vi "ClientSrv Remote File Dialog.vi"(7 "prompt":string, 8 "pattern":string(combo), 11 "start path":path) -> (0 "cancelled":bool, 2 "path":path)   [LabVIEW 2012]
doc: "A file dialog for selecting a file on the remote server. Can be called as a subVI similar to the standard \"File Dialog\" function."
uses:
  served/ClientSrv Server File Manipulation_srv.ctl
  typedefs/t_ClientSrv Remote File Dialog States.ctl
  typedefs/t_ClientSrv Tree Controller Methods.ctl
panel:
  out "file manipulation":T1
  out "file":string
  in  "cancel":bool
  in  "select":bool
  in  "tree":string(tree)
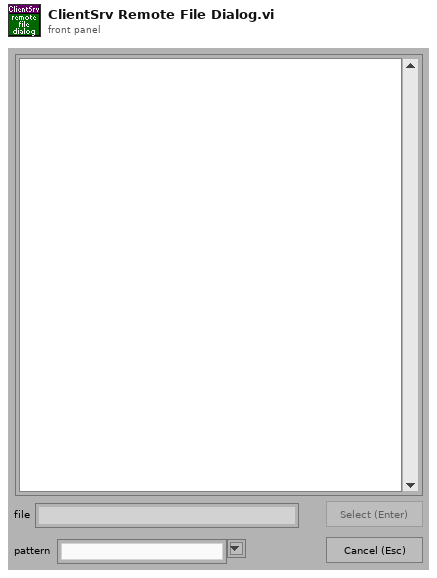
[diagram p1: front panel]
types:
  T1 = typedef "ClientSrv Server File Manipulation_srv.ctl" = refnum<vi>
  T2 = typedef "t_ClientSrv Remote File Dialog States.ctl" = enum16{"empty queue", "initialize", "update tree", "update selected", "persist", "cleanup", "stop"}
  T3 = typedef "t_ClientSrv Tree Controller Methods.ctl" = enum16{"do nothing", "initialize", "open item", "close item", "refresh"}
  T4 = typedef "eventvkey.ctl" = enum16{"ASCII", "Enter", "Return", "Shift", "Ctrl", "Alt", "Cmd", "Opt", "Caps", "NumLock", "Clear", "Break", "Up", "Down", "Left", "Right", "Insert", "Delete", "Home", "End", "PageUp", "PageDown", "Escape", "Help", "Pause", "ScrollLock", "F1", "F2", "F3", "F4", "F5", "F6", "F7", "F8", "F9", "F10", "F11", "F12", "F13", "F14", "F15", "F16", "F17", "F18", "F19", "F20", "F21", "F22", "F23", "F24", "Play", "VolumeUp", "VolumeDown", "Mute", "Two Byte Char"}
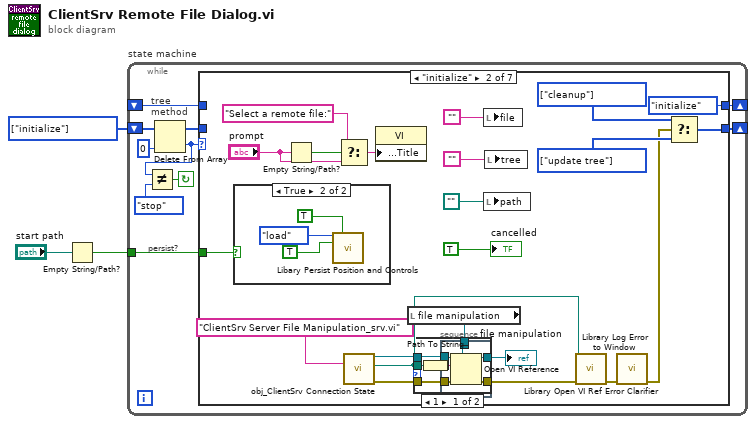
[diagram p0: block diagram]
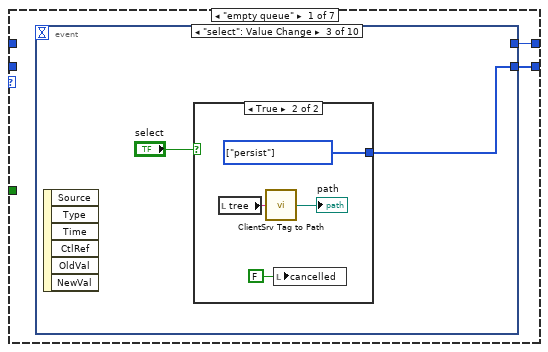
[diagram p2: hidden frame]
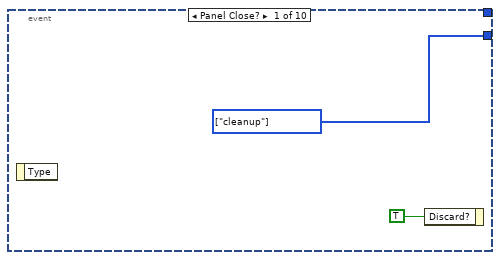
[diagram p3: hidden frame]
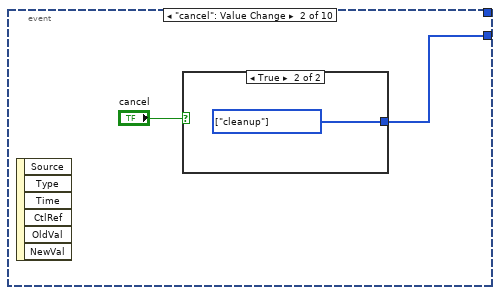
[diagram p4: hidden frame]
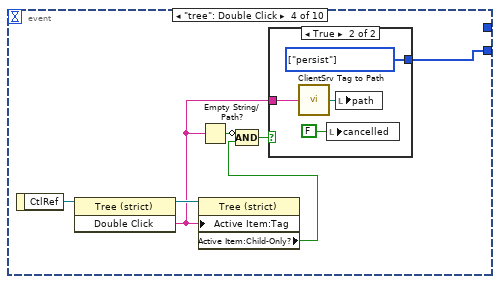
[diagram p7: hidden frame]
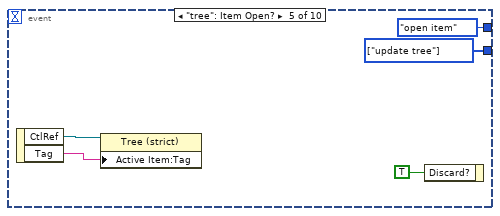
[diagram p9: hidden frame]
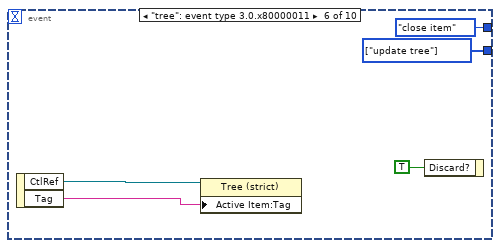
[diagram p10: hidden frame]
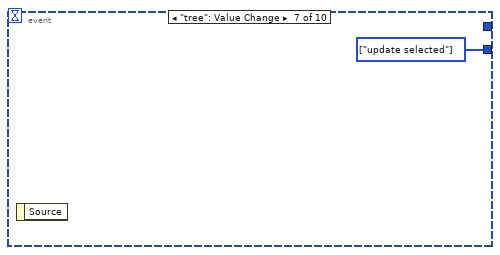
[diagram p11: hidden frame]
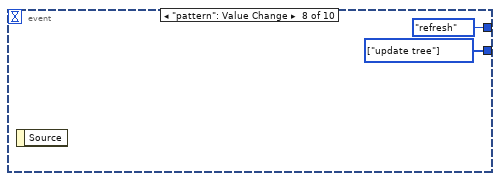
[diagram p12: hidden frame]
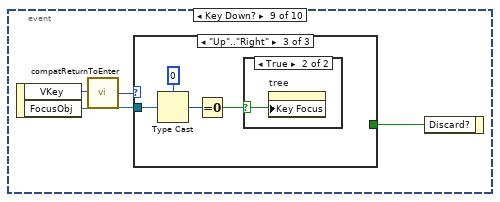
[diagram p13: hidden frame]
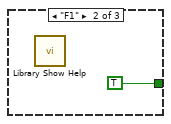
[diagram p15: hidden frame]
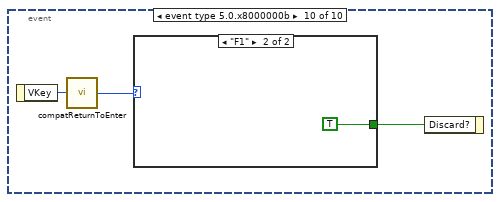
[diagram p17: hidden frame]
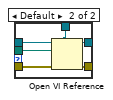
[diagram p19: hidden frame]
diagram:
  w3 = T2[] [enum."initialize"] items=["empty queue", "initialize", "update tree", "update selected", "persist", "cleanup", "stop"] ("Array Constant")
  n1 = Empty String/Path?(string/path="start path") -> (empty?=w1:bool)
  n2 = while "state machine" {
    shift-left: w3 -> [w10]
    shift-right: [w13] -> _
    shift-right: [w5] -> _
    shift-left: _ -> [w6]
    tunnel: w1 -> [w4]
    stop <- w12 continue-if-true
    # "persist?"
    # "tree\nmethod"
    n3 = Delete From Array(array=w10, index=0) -> (deleted portion=w8:T2, array with subset deleted=w9:T2[])  [unwired: 1 in]
    n4 = Not Equal?(x=w8, y=t_ClientSrv_Remote_File_Dialog_States."stop" ("states")) -> (x != y?=w12:bool)
    n5 = case "Case" shown="\"initialize\"" w8 {
      tunnel: [w15 w75 w112 w129 w137 w150 w152] -> w13
      tunnel: w9 -> [_ _ w114 w129 w139 _ w152]
      tunnel: w6 -> [_ _ w113 w128 w138 w149 w151]
      tunnel: [w14 t_ClientSrv_Tree_Controller_Methods."initialize" ("method") w113 w128 w138 w149 w151] -> w5
      tunnel: w4 -> [_ w71 _ _ w135 _ _]
      frame "empty queue" {
        n6 = event shown="[2] \"select\": Value Change" {
          selector: _ -> [_ _ _ _ _ _ _ _ _ _]
          dyn-events: _ -> [_ _ _ _ _ _ _ _ _ _]
          timeout: _ -> [_ _ _ _ _ _ _ _ _ _]
          tunnel: [w17 w19 w22 w29 w42 w45 w48 w49 _ _] -> w15
          tunnel: [_ _ _ _ t_ClientSrv_Tree_Controller_Methods."open item" ("method") t_ClientSrv_Tree_Controller_Methods."close item" ("method") _ t_ClientSrv_Tree_Controller_Methods."refresh" ("method") _ _] -> w14
          event Panel Close? {
            w17 = T2[] [enum."cleanup"] items=["empty queue", "initialize", "update tree", "update selected", "persist", "cleanup", "stop"] ("Array Constant")
            n7 = event-data() -> ()  [unwired: 1 in, 1 out]
            n8 = event-data("Discard?"=TRUE) -> ()  [unwired: 1 in, 1 out]
          }
          event "cancel": Value Change {
            n9 = event-data() -> ()  [unwired: 1 in, 6 out]
            n10 = case shown="True" "cancel" {
              tunnel: [_ w20] -> w19
              frame False {
              }
              frame True {
                w20 = T2[] [enum."cleanup"] items=["empty queue", "initialize", "update tree", "update selected", "persist", "cleanup", "stop"] ("Array Constant")
              }
            }
          }
          event "select": Value Change {
            n11 = event-data() -> ()  [unwired: 1 in, 6 out]
            n12 = case shown="True" "select" {
              tunnel: [_ w26] -> w22
              frame False {
              }
              frame True {
                w26 = T2[] [enum."persist"] items=["empty queue", "initialize", "update tree", "update selected", "persist", "cleanup", "stop"] ("Array Constant")
                n13 = local read "tree"() -> (w25:string)
                n14 = call "ClientSrv Tag to Path.vi"("tree tag"=w25) -> ("path"=→"path":path)
                n15 = local write "cancelled"(FALSE ("cancelled")) -> ()
              }
            }
          }
          event "tree": Double Click {
            n16 = event-data() -> ("CtlRef"=w33:refnum<vi>)  [unwired: 1 in]
            n17 = invoke class="Tree (strict)" method="Double Click"(reference=w33) -> (reference out=w32:refnum<vi>, "Double Click"=w27:string)  [unwired: 2 in, 1 out]
            n18 = property class="Tree (strict)"(reference=w32, "Active Item:Tag"=w27) -> ("Active Item:Child-Only?"=w28:bool)  [unwired: 1 in, 2 out]
            n19 = Empty String/Path?(string/path=w27) -> (empty?=w31:bool)
            n20 = Compound Arithmetic op=AND(invert w31, w28) -> (w30:bool)
            n21 = case shown="True" w30 {
              tunnel: w27 -> [_ w36]
              tunnel: [_ w35] -> w29
              frame False {
              }
              frame True {
                w35 = T2[] [enum."persist"] items=["empty queue", "initialize", "update tree", "update selected", "persist", "cleanup", "stop"] ("Array Constant")
                n22 = call "ClientSrv Tag to Path.vi"("tree tag"=w36) -> ("path"=w37:path)
                n23 = local write "cancelled"(FALSE ("cancelled")) -> ()
                n24 = local write "path"(w37) -> ()
              }
            }
          }
          event "tree": Item Open? {
            w42 = T2[] [enum."update tree"] items=["empty queue", "initialize", "update tree", "update selected", "persist", "cleanup", "stop"] ("Array Constant")
            n25 = event-data() -> ("CtlRef"=w41:refnum<vi>, "Tag"=w40:string)  [unwired: 1 in]
            n26 = property class="Tree (strict)"(reference=w41, "Active Item:Tag"=w40) -> ()  [unwired: 1 in, 2 out]
            n27 = event-data("Discard?"=TRUE) -> ()  [unwired: 1 in, 1 out]
          }
          event "tree": event type 3.0.x80000011 {
            w45 = T2[] [enum."update tree"] items=["empty queue", "initialize", "update tree", "update selected", "persist", "cleanup", "stop"] ("Array Constant")
            n28 = event-data() -> ("CtlRef"=w47:refnum<vi>, "Tag"=w46:string)  [unwired: 1 in]
            n29 = property class="Tree (strict)"(reference=w47, "Active Item:Tag"=w46) -> ()  [unwired: 1 in, 2 out]
            n30 = event-data("Discard?"=TRUE) -> ()  [unwired: 1 in, 1 out]
          }
          event "tree": Value Change {
            w48 = T2[] [enum."update selected"] items=["empty queue", "initialize", "update tree", "update selected", "persist", "cleanup", "stop"] ("Array Constant")
            n31 = event-data() -> ()  [unwired: 1 in, 1 out]
          }
          event "pattern": Value Change {
            w49 = T2[] [enum."update tree"] items=["empty queue", "initialize", "update tree", "update selected", "persist", "cleanup", "stop"] ("Array Constant")
            n32 = event-data() -> ()  [unwired: 1 in, 1 out]
          }
          event Key Down? {
            n33 = event-data() -> ("VKey"=w51:T4, "FocusObj"=w52:refnum<vi>)  [unwired: 1 in]
            n34 = call <vilib>:"compatReturnToEnter.vi"("VKey"=w51) -> ("VKey"=w54:T4)
            n35 = case shown="\"Up\"..\"Right\"" w54 {
              tunnel: [_ TRUE _] -> w53
              tunnel: w52 -> [_ _ w57]
              frame Default {
              }
              frame "F1" {
                n36 = call "Library Show Help.vi"() -> ()  [unwired: 1 in]
              }
              frame "Up".."Right" {
                n37 = Type Cast(type=0, x=w57) -> (*(type *) &x=w59:i32)
                n38 = Equal To 0?(x=w59) -> (x = 0?=w56:bool)
                n39 = case shown="True" w56 {
                  selector: w56 -> [_ w60]
                  frame False {
                  }
                  frame True {
                    n40 = property on="tree" class="Tree (strict)"("Key Focus"=w60) -> ()  [unwired: 2 in, 2 out]
                  }
                }
              }
            }
            n41 = event-data("Discard?"=w53) -> ()  [unwired: 1 in, 1 out]
          }
          event event type 5.0.x8000000b {
            n42 = event-data() -> ("VKey"=w61:T4)  [unwired: 1 in]
            n43 = call <vilib>:"compatReturnToEnter.vi"("VKey"=w61) -> ("VKey"=w63:T4)
            n44 = case shown="\"F1\"" w63 {
              tunnel: [_ TRUE] -> w62
              frame Default {
              }
              frame "F1" {
              }
            }
            n45 = event-data("Discard?"=w62) -> ()  [unwired: 1 in, 1 out]
          }
        }
      }
      frame "initialize" {
        w74 = T2[] [enum."cleanup"] items=["empty queue", "initialize", "update tree", "update selected", "persist", "cleanup", "stop"] ("Array Constant")
        w73 = T2[] [enum."update tree"] items=["empty queue", "initialize", "update tree", "update selected", "persist", "cleanup", "stop"] ("Array Constant")
        n46 = case shown="True" w71 {
          frame False {
          }
          frame True {
            n47 = call "Libary Persist Position and Controls.vi"("action"=enum16{"save", "load"}."load", "do not open (false)"=TRUE, "do not persist bounds (false)"=TRUE) -> ()  [unwired: 11 in, 2 out]
          }
        }
        n48 = Empty String/Path?(string/path="prompt") -> (empty?=w81:bool)
        n49 = Select(t="Select a remote file:", s=w81, f="prompt") -> (s? t:f=w78:string)
        n50 = call "obj_ClientSrv Connection State.vi"("machine{connect}/VI{get state} name (local/no path resolution)"="ClientSrv Server File Manipulation_srv.vi") -> ("server app ref"=w66:refnum<vi>, "resolved server path"=w65:path, "error out"=w70:errorcluster)  [unwired: 7 in, 5 out]
        n51 = property class="VI"("Front Panel Window:Title"=w78) -> ()  [unwired: 2 in, 2 out]
        n52 = local read "file manipulation"() -> (w67:T1)
        n53 = stacked-sequence {
          tunnel: [w92] -> w68
          tunnel: [w91] -> w69
          tunnel: w70 -> [w90]
          tunnel: w66 -> [w89]
          tunnel: w65 -> [w88]
          tunnel: w67 -> [w87]
          frame #0 {
            # "avoid LV8 complaints"
            n54 = Path to Array of Strings(0:w88) -> (2:w93:string[])  [unwired: 1 out]
            n55 = Array Size(array=w93) -> (size(s)=w94:i32)
            n56 = case shown="1" w94 {
              tunnel: w88 -> [w101 w107]
              tunnel: w89 -> [w99 w106]
              tunnel: [w97 w102] -> w92
              tunnel: [w95 w105] -> w91
              tunnel: w87 -> [w96 w104]
              tunnel: w90 -> [w98 w103]
              frame 1 {
                n57 = Path To String(path=w101) -> (string=w100:string)
                n58 = Open VI Reference(type specifier VI Refnum (for type only)=w96, application reference (local)=w99, vi path=w100, error in (no error)=w98) -> (vi reference=w97:T1, error out=w95:errorcluster)  [unwired: 2 in]
              }
              frame Default {
                n59 = Open VI Reference(type specifier VI Refnum (for type only)=w104, application reference (local)=w106, vi path=w107, error in (no error)=w103) -> (vi reference=w102:T1, error out=w105:errorcluster)  [unwired: 2 in]
              }
            }
          }
        }
        "file manipulation" <- w68
        n60 = local write "file"("") -> ()
        n61 = local write "path"(path "") -> ()
        n62 = local write "tree"("") -> ()
        n63 = call "Library Open VI Ref Error Clarifier.vi"("VI path"=w65, "called VI error (no error)"=w69) -> ("error out"=w76:errorcluster)  [unwired: 13 in]
        n64 = call "Library Log Error to Window.vi"("error in (no error)"=w76) -> ("dup error"=w72:errorcluster)  [unwired: 13 in, 1 out]
        n65 = Select(t=w74, s=w72, f=w73) -> (s? t:f=w75:T2[])
        "cancelled" <- TRUE ("cancelled")
      }
      frame "update tree" {
        n66 = flat-sequence {
          tunnel: w113 -> [w121]
          frame #0 {
            n67 = property class="VI"() -> ("Front Panel"=w116:refnum<vi>)  [unwired: 2 in, 2 out]
            n68 = call <vilib>:"Set Busy.vi"() -> ()  [unwired: 10 in, 2 out]
            n69 = property class="Pnl"(reference=w116, "Defer Panel Updates"=TRUE) -> ()  [unwired: 1 in, 2 out]
          }
          frame #1 {
            n70 = control-ref of="tree"() -> (w119:refnum<vi>)
            n71 = local read "start path"() -> (w117:path)
            n72 = local read "file manipulation"() -> (w120:T1)
            n73 = call "re_ClientSrv Tree Controller.vi"("method"=w121, "start path"=w117, "tree control reference"=w119, "pattern"="pattern", "file manipulation (local)"=w120) -> ()  [unwired: 11 in]
          }
          frame #2 {
            n74 = property class="VI"() -> ("Front Panel"=w123:refnum<vi>)  [unwired: 2 in, 2 out]
            n75 = property class="Pnl"(reference=w123, "Defer Panel Updates"=FALSE) -> ()  [unwired: 1 in, 2 out]
            n76 = call <vilib>:"Unset Busy.vi"() -> ()  [unwired: 11 in, 1 out]
          }
        }
        n77 = Build Array (concatenate)(t_ClientSrv_Remote_File_Dialog_States."update selected" ("states"), w114) -> (w112:T2[])
      }
      frame "update selected" {
        n78 = property on="tree" class="Tree (strict)"("Active Item:Tag"="tree") -> ("Active Item:Child-Only?"=w126:bool)  [unwired: 2 in, 2 out]
        n79 = case shown="True" w126 {
          tunnel: "tree" -> [_ w133]
          tunnel: [w130 w134] -> w125
          tunnel: [_ w131] -> w124
          frame False {
            w130 = u8 2 items=["enabled", "disabled", "grayed"] ("disabled state")
          }
          frame True {
            w134 = u8 0 items=["enabled", "disabled", "grayed"] ("disabled state")
            n80 = call "ClientSrv Tag to Path.vi"("tree tag"=w133) -> ("path"=w132:path)
            n81 = Strip Path(path=w132) -> (name=w131:string)  [unwired: 1 out]
          }
        }
        "file" <- w124
        n82 = property on="select" class="Bool"("Disabled"=w125) -> ()  [unwired: 2 in, 2 out]
      }
      frame "persist" {
        n83 = case shown="True" w135 {
          frame False {
          }
          frame True {
            n84 = flat-sequence {
              frame #0 {
                n85 = local read "path"() -> (w141:path)
                n86 = Strip Path(path=w141) -> (stripped path=w140:path)  [unwired: 1 out]
                n87 = local write "start path"(w140) -> ()
              }
              frame #1 {
                n88 = call "Libary Persist Position and Controls.vi"("action"=enum16{"save", "load"}."save", "do not persist bounds (false)"=TRUE) -> ()  [unwired: 12 in, 2 out]
              }
            }
          }
        }
        n89 = Build Array (concatenate)(t_ClientSrv_Remote_File_Dialog_States."cleanup" ("states"), w139) -> (w137:T2[])
      }
      frame "cleanup" {
        w150 = T2[] [enum."stop"] items=["empty queue", "initialize", "update tree", "update selected", "persist", "cleanup", "stop"] ("Array Constant")
        n90 = local read "file manipulation"() -> (w145:T1)
        n91 = invoke on="tree" class="TreeControl (strict)" method="Edit Tree Items.Delete"("Delete Children"=TRUE) -> ()  [unwired: 4 in, 5 out]
        n92 = local write "file"("") -> ()
        n93 = local write "pattern"("") -> ()
        n94 = local write "start path"(path "") -> ()
        n95 = Close Reference(reference=w145) -> ()  [unwired: 1 in, 1 out]
      }
      frame "stop" {
      }
    }
  }
